vi "Export.vi"(8 "error in (no error)":errorcluster, 11 "DataBase in":refnum<class "DataBase.lvclass">) -> (0 "error out":errorcluster, 3 "DataBase out":refnum<class "DataBase.lvclass">)   [LabVIEW 2019, in "DataBase.lvlib" / "DataBase.lvclass"]
uses:
  DataBase.lvclass
  DataBase.lvclass/DataBase.ctl
  <vilib>/Utility/NIReport.llb/Report Type.ctl
  <vilib>/addons/_office/excel.llb/Excel Easy Table (str).vi
  <vilib>/Utility/NIReport.llb/NI_report.lvclass
  <vilib>/addons/_office/NI_ReportGenerationToolkit.lvlib
  <vilib>/Utility/NIReport.llb/NI_ReportGenerationCore.lvlib
panel:
  in  "Radio Buttons":enum32{"CSV", "PDF", "Excel", "XML"}(radio)
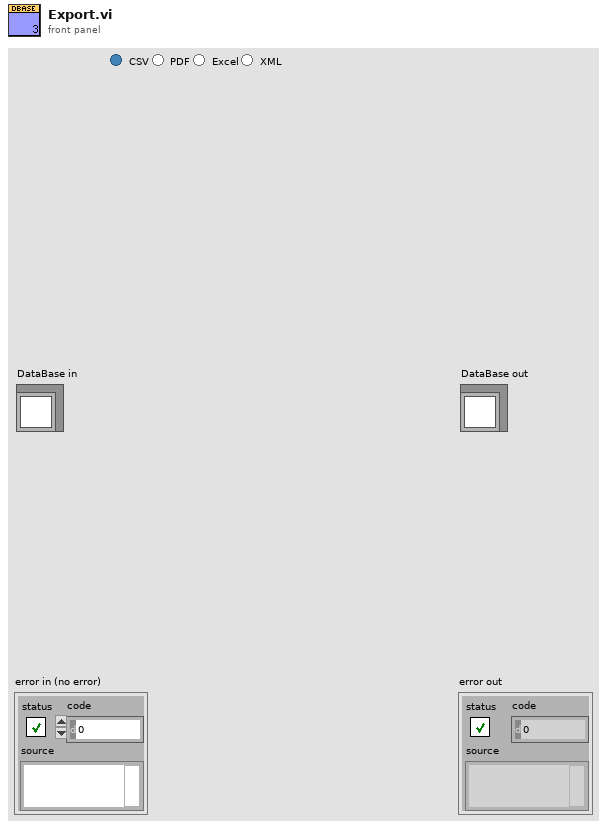
[diagram p1: front panel]
types:
  T1 = typedef "NI_ReportGenerationCore.lvlib/Report Type.ctl" = enum16{"HTML", "Word", "Excel"}
  T2 = enum16{"maximized", "minimized", "normal", "no change"}
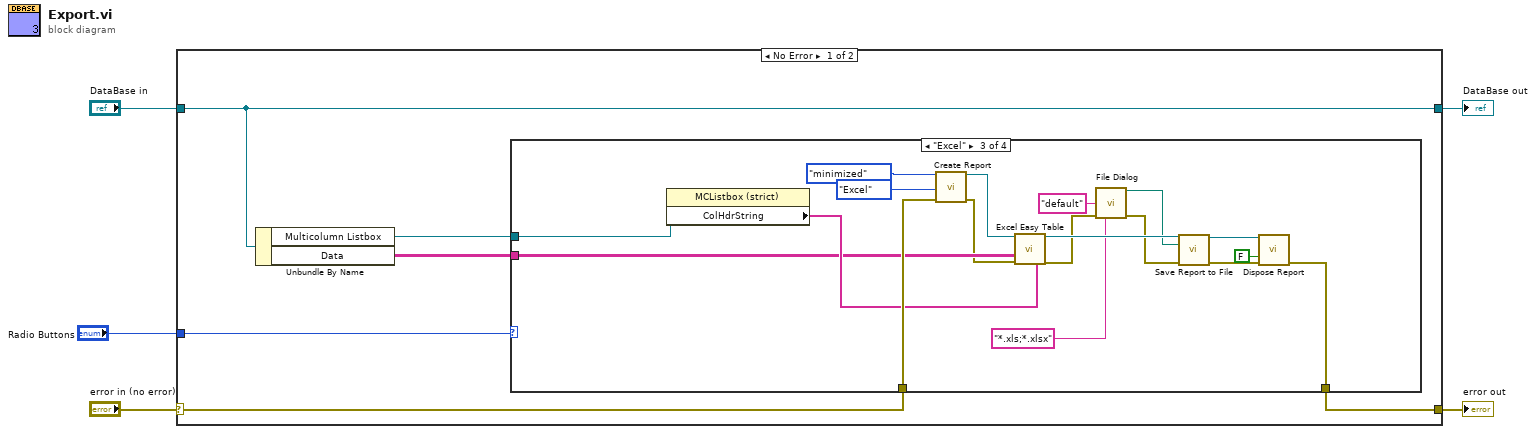
[diagram p0: block diagram]
diagram:
  n1 = case shown="No Error" "error in (no error)" {
    selector: "error in (no error)" -> [w10 w34]
    tunnel: [w9 w34] -> w4
    tunnel: [w11 w33] -> w2
    tunnel: "DataBase in" -> [w11 w33]
    tunnel: "Radio Buttons" -> [w6 _]
    frame No Error {
      n2 = Unbundle By Name(w11) -> ("Multicolumn Listbox"=w8:refnum<vi>, "Data"=w7:string[][])
      n3 = case shown="\"Excel\"" w6 {
        tunnel: w10 -> [w12 w13 w31 w32]
        tunnel: [w12 w13 w30 w32] -> w9
        tunnel: w8 -> [_ _ w29 _]
        tunnel: w7 -> [_ _ w27 _]
        frame "CSV", Default {
        }
        frame "PDF" {
        }
        frame "Excel" {
          n4 = property class="MCListbox (strict)"(reference=w29) -> ("ColHdrString"=w28:string[])  [unwired: 1 in, 2 out]
          n5 = call <vilib>:"Create Report.vi"("window state (normal)"=T2."minimized", "report type"=Report_Type."Excel", "error in (no error)"=w31) -> ("report out"=w24:refnum<class "NI_report.lvclass">, "error out"=w23:errorcluster)  [unwired: 11 in]
          n6 = call-poly <vilib>:"Excel Easy Table.vi"("report in"=w24, "text data"=w27, "error in (no error)"=w23, "column headers"=w28) -> ("report out"=w22:refnum<class "NI_report.lvclass">, "error out"=w17:errorcluster)  [unwired: 7 in, 3 out]
          n7 = call "File Dialog"("default name"="default", "error in"=w17, "pattern (all files)"="*.xls;*.xlsx") -> ("selected path"=w18:path, "error out"=w16:errorcluster)  [unwired: 9 in, 2 out]
          n8 = call-dynamic "Save Report to File.vi"("report in"=w22, "report file path"=w18, "error in (no error)"=w16) -> ("report out"=w21:refnum<class "NI_report.lvclass">, "error out"=w20:errorcluster)  [unwired: 11 in]
          n9 = call-dynamic "Dispose Report.vi"("report in"=w21, "save changes? (F)"=FALSE, "error in (no error)"=w20) -> ("error out"=w30:errorcluster)  [unwired: 12 in]
        }
        frame "XML" {
        }
      }
    }
    frame Error {
    }
  }
  "error out" <- w4
  "DataBase out" <- w2
